vi "8-Test PingReq NoIdentifier.vi"() -> ()   [LabVIEW 2013]
uses:
  <vilib>/LabVIEW Open Source Project/MQTT Connection/MQTT_Connection/Connection/Connection.lvclass/Connection.ctl
  source/Server class/Server.lvclass/Server.ctl
  <vilib>/LabVIEW Open Source Project/MQTT Client/Client class/Client.lvclass/Client.ctl
  <vilib>/LabVIEW Open Source Project/MQTT Control Packets/Control Packets/PUBLISH/PUBLISH.lvclass
  source/Server class/Server.lvclass
  <vilib>/LabVIEW Open Source Project/MQTT Connection/MQTT_Base/Base Class/MQTT_Base.lvclass
  <vilib>/LabVIEW Open Source Project/MQTT Client/Client class/Client.lvclass
  <vilib>/LabVIEW Open Source Project/MQTT TCP Connection/MQTT_TCP/Connection/TCPConnection.lvclass
  <vilib>/LabVIEW Open Source Project/MQTT LocalQueue Connection/MQTT_LocalQueue/Connection/LocalQueueConnection.lvclass
  <vilib>/LabVIEW Open Source Project/MQTT Connection/MQTT_Connection/Connection/Connection.lvclass
  <vilib>/LabVIEW Open Source Project/MQTT Connection/MQTT_Base/DebuggingTerminal/DebuggingTerminal.lvclass
panel:
  out "#publish":i32
  out "error client source 2":errorcluster
  out "Published":bool
  out "ping time":i32
  out "#pings":i32
  out "PING FAILURE":bool
  out "Server responded":bool
  out "error server":errorcluster
  out "error client source":errorcluster
  out "NbConnections":u32
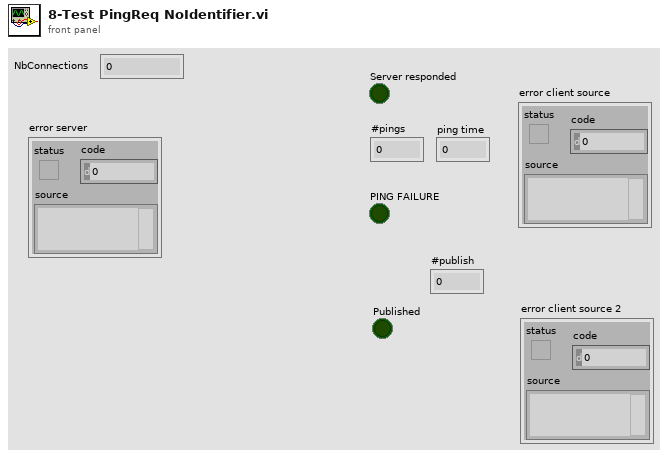
[diagram p1: front panel]
types:
  T1 = typedef "MQTT Client.lvlib/Client.lvclass/Public Events -- cluster.ctl" = cluster{"Connection Status":refnum<user-event>, "Connected":refnum<user-event>, "Application Message":refnum<user-event>}
  T2 = typedef "MQTT Server.lvlib/Server.lvclass/Public Events -- cluster.ctl" = cluster{"NbConnections":refnum<user-event>, "Client Event":refnum<user-event>}
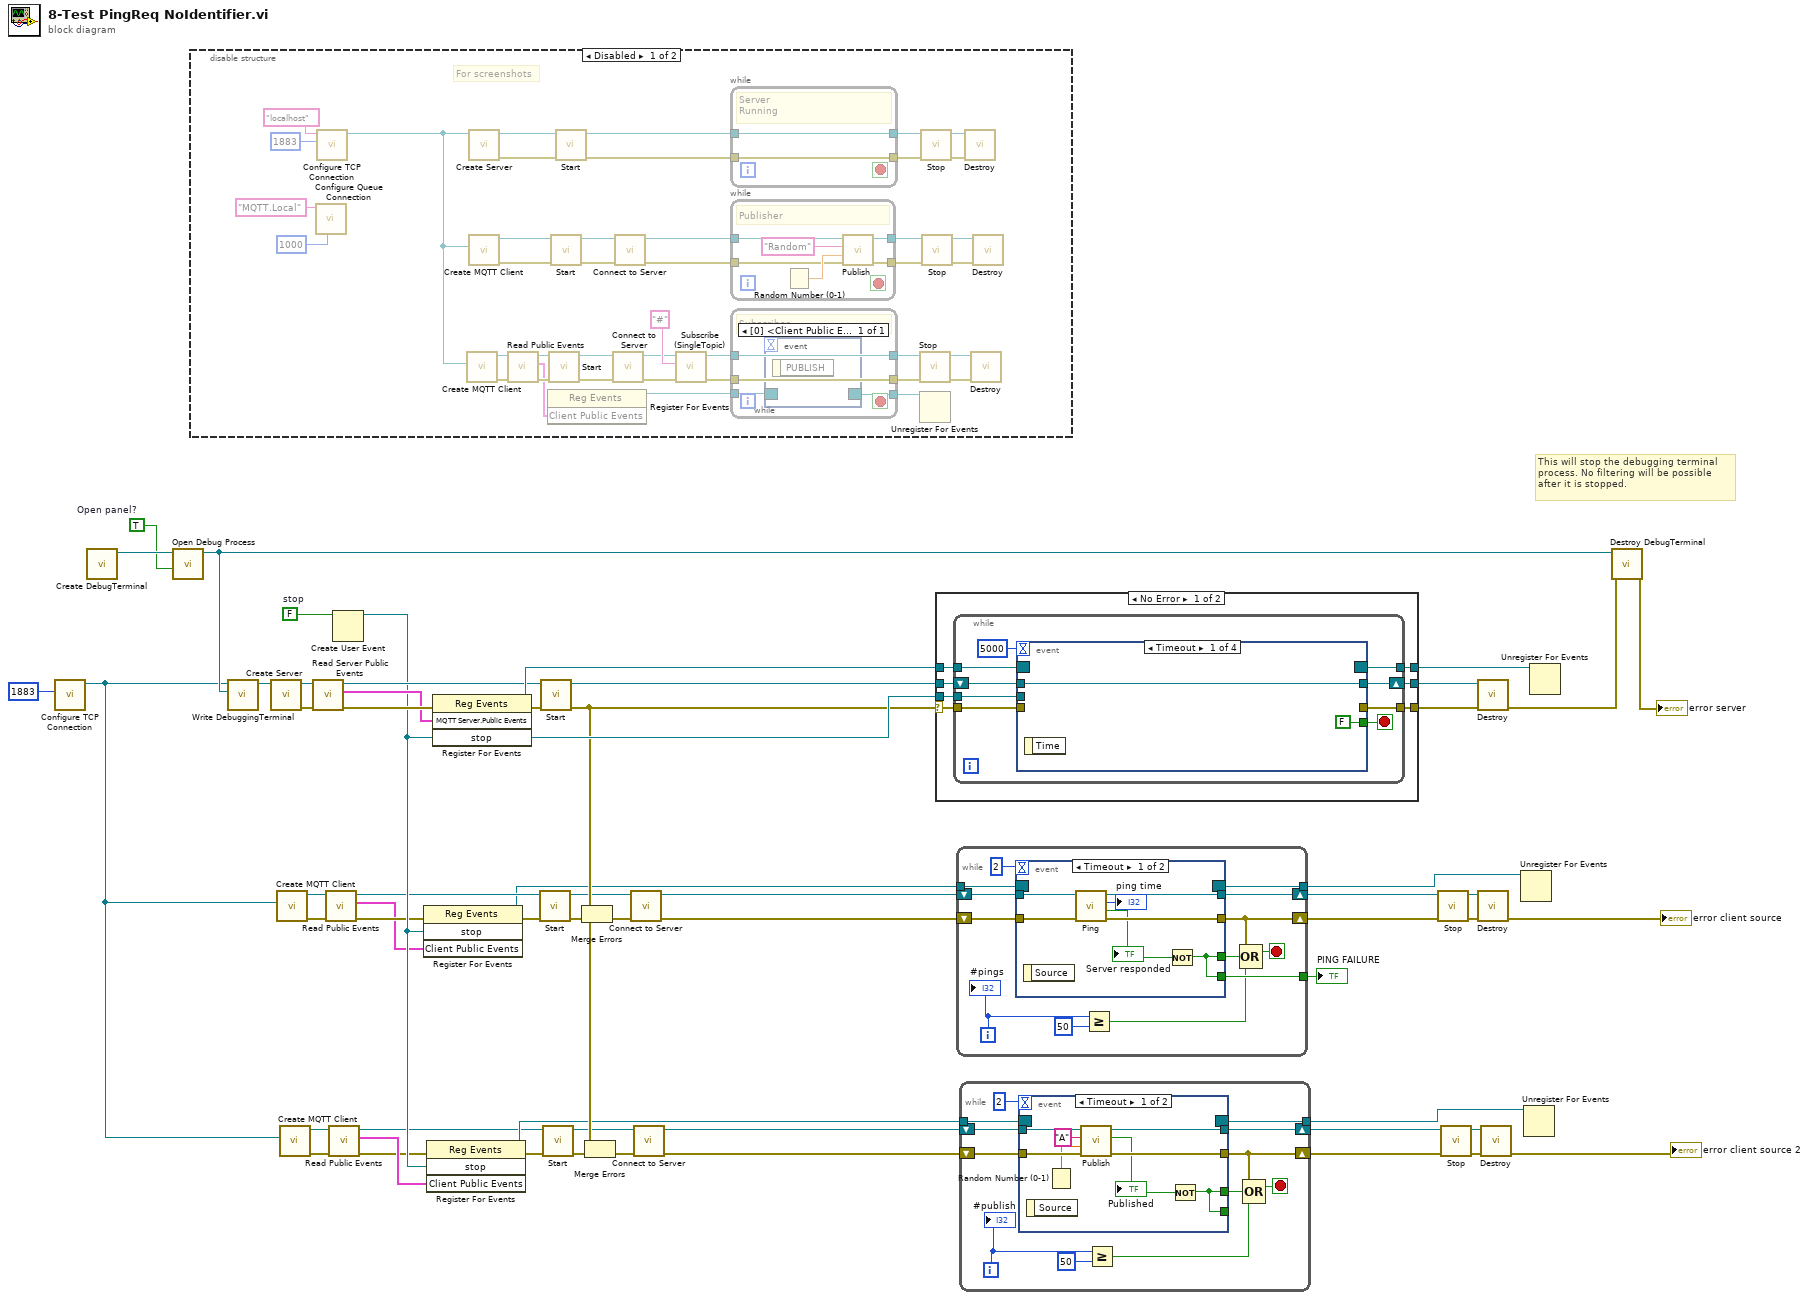
[diagram p0: block diagram]
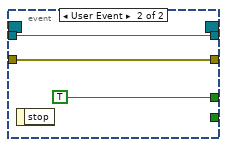
[diagram p2: hidden frame]
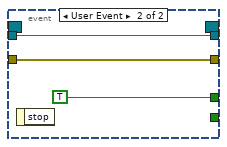
[diagram p3: hidden frame]
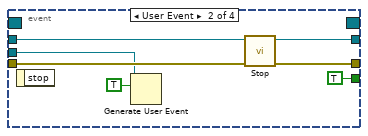
[diagram p5: hidden frame]
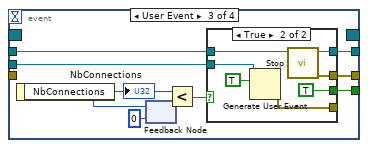
[diagram p6: hidden frame]
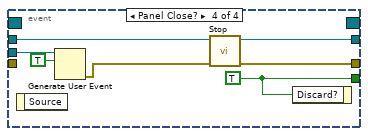
[diagram p8: hidden frame]
diagram:
  w1 = TRUE  # Open panel?
  w48 = FALSE  # stop
  # "This will stop the debugging terminal\nprocess. No filtering will be possible\nafter it is stopped."
  n1 = call <vilib>:"Configure TCP Connection.vi"("remote port (80)"=u16 1883) -> ("TCPConnection"=w5:refnum<class "TCPConnection.lvclass">)  [unwired: 9 in, 1 out]
  n2 = call <vilib>:"Create DebugTerminal.vi"() -> ("DebuggingTerminal out"=w9:refnum<class "DebuggingTerminal.lvclass">)  [unwired: 10 in, 1 out]
  n3 = call <vilib>:"Open Debug Process.vi"("Open panel?"=w1, "DebuggingTerminal in"=w9) -> ("DebuggingTerminal out"=w7:refnum<class "DebuggingTerminal.lvclass">)  [unwired: 8 in, 1 out]
  n4 = disable-structure shown="Disabled" {
    frame Disabled {
      # "For screenshots"
      n5 = call <vilib>:"Configure Queue Connection.vi"("timeout (500 ms)"=1000 ("timeout (100ms)"), "Queue Name"="MQTT.Local") -> ()  [unwired: 8 in, 2 out]
      n6 = call <vilib>:"Configure TCP Connection.vi"("remote port (80)"=u16 1883, "address (localhost)"="localhost" ("Topic Filter")) -> ("TCPConnection"=w63:refnum<class "TCPConnection.lvclass">)  [unwired: 8 in, 1 out]
      n7 = call <vilib>:"Create MQTT Client.vi"("Connection Configuration"=w63) -> ("error out"=w69:errorcluster, "Client out"=w71:refnum<class "Client.lvclass">)  [unwired: 9 in]
      n8 = call "Create Server.vi"("Connection Configuration"=w63) -> ("error out"=w94:errorcluster, "Server"=w93:refnum<class "Server.lvclass">)  [unwired: 9 in]
      n9 = call <vilib>:"Create MQTT Client.vi"("Connection Configuration"=w63) -> ("error out"=w91:errorcluster, "Client out"=w92:refnum<class "Client.lvclass">)  [unwired: 9 in]
      n10 = call <vilib>:"Read Public Events.vi"("error in (no error)"=w69, "Client in"=w71) -> ("error out"=w68:errorcluster, "Client Public Events"=w67:T1, "Client out"=w70:refnum<class "Client.lvclass">)  [unwired: 7 in]
      n11 = register-events(w67) -> (reference out=w66:refnum<event-registration>)  [unwired: 2 in, 1 out]
      n12 = call <vilib>:"Start.vi"("error in (no error)"=w68, "MQTT_Base in"=w70) -> ("error out"=w86:errorcluster, "MQTT_Base out"=w87:refnum<class "Client.lvclass">)  [unwired: 7 in, 1 out]
      n13 = call <vilib>:"Start.vi"("error in (no error)"=w91, "MQTT_Base in"=w92) -> ("error out"=w98:errorcluster, "MQTT_Base out"=w97:refnum<class "Client.lvclass">)  [unwired: 7 in, 1 out]
      n14 = call <vilib>:"Start.vi"("error in (no error)"=w94, "MQTT_Base in"=w93) -> ("error out"=w78:errorcluster, "MQTT_Base out"=w80:refnum<class "Server.lvclass">)  [unwired: 7 in, 1 out]
      n15 = call <vilib>:"Connect to Server.vi"("error in (no error)"=w86, "Client in"=w87) -> ("error out"=w74:errorcluster, "Client out"=w75:refnum<class "Client.lvclass">)  [unwired: 6 in, 2 out]
      n16 = call <vilib>:"Connect to Server.vi"("error in (no error)"=w98, "Client in"=w97) -> ("error out"=w82:errorcluster, "Client out"=w85:refnum<class "Client.lvclass">)  [unwired: 6 in, 2 out]
      n17 = call <vilib>:"Subscribe (SingleTopic).vi"("error in (no error)"=w74, "Topic Filter"="#", "MQTT_Base in"=w75) -> ("error out"=w72:errorcluster, "MQTT_Base out"=w73:refnum<class "Client.lvclass">)  [unwired: 6 in, 1 out]
      n18 = while {
        tunnel: [w112] -> w81
        tunnel: w80 -> [w112]
        tunnel: w78 -> [w111]
        tunnel: [w111] -> w79
        stop <- _ stop-if-true
        # "Server\nRunning"
      }
      n19 = while {
        tunnel: w85 -> [w108]
        tunnel: [w107] -> w84
        tunnel: [w106] -> w83
        tunnel: w82 -> [w105]
        stop <- _ stop-if-true
        # "Publisher"
        n20 = Random Number (0-1)() -> (number: 0 to 1=w110:dbl)
        n21 = call <vilib>:"Publish.vi"("error in (no error)"=w105, "Payload"=w110, "Topic Name (empty: Payload name)"="Random", "Client in"=w108) -> ("error out"=w106:errorcluster, "Client out"=w107:refnum<class "Client.lvclass">)  [unwired: 5 in, 1 out]
      }
      n22 = while {
        tunnel: [w104] -> w76
        tunnel: w73 -> [w104]
        tunnel: w72 -> [w103]
        tunnel: [w103] -> w77
        tunnel: w66 -> [w102]
        tunnel: [w101] -> w65
        stop <- _ stop-if-true
        # "Subscriber"
        n23 = event shown="[0] <Client Public Events.Application Message>: User Event" {
          selector: w102 -> [_]
          dyn-events: [_] -> w101
          timeout: _ -> [_]
          event User Event {
            n24 = event-data() -> ()  [unwired: 1 in, 1 out]
          }
        }
      }
      n25 = call <vilib>:"Stop.vi"("error in (no error)"=w77, "MQTT_Base in"=w76) -> ("error out"=w89:errorcluster, "MQTT_Base out"=w90:refnum<class "Client.lvclass">)  [unwired: 7 in, 1 out]
      n26 = Unregister For Events(event registration refnum=w65) -> ()  [unwired: 1 in, 1 out]
      n27 = call <vilib>:"Stop.vi"("error in (no error)"=w79, "MQTT_Base in"=w81) -> ("error out"=w100:errorcluster, "MQTT_Base out"=w99:refnum<class "Server.lvclass">)  [unwired: 7 in, 1 out]
      n28 = call <vilib>:"Stop.vi"("error in (no error)"=w83, "MQTT_Base in"=w84) -> ("error out"=w96:errorcluster, "MQTT_Base out"=w95:refnum<class "Client.lvclass">)  [unwired: 7 in, 1 out]
      n29 = call <vilib>:"Destroy.vi"("error in (no error)"=w100, "MQTT_Base in"=w99) -> ()  [unwired: 8 in, 2 out]
      n30 = call <vilib>:"Destroy.vi"("error in (no error)"=w89, "MQTT_Base in"=w90) -> ()  [unwired: 8 in, 2 out]
      n31 = call <vilib>:"Destroy.vi"("error in (no error)"=w96, "MQTT_Base in"=w95) -> ()  [unwired: 8 in, 2 out]
    }
    frame Enabled {
    }
  }
  n32 = call <vilib>:"Write DebuggingTerminal.vi"("DebuggingTerminal"=w7, "Connection in"=w5) -> ("Connection out"=w4:refnum<class "TCPConnection.lvclass">)  [unwired: 9 in]
  n33 = call "Create Server.vi"("Connection Configuration"=w4) -> ("error out"=w57:errorcluster, "Server"=w58:refnum<class "Server.lvclass">)  [unwired: 9 in]
  n34 = call <vilib>:"Create MQTT Client.vi"("Connection Configuration"=w5) -> ("error out"=w44:errorcluster, "Client out"=w43:refnum<class "Client.lvclass">)  [unwired: 9 in]
  n35 = call <vilib>:"Create MQTT Client.vi"("Connection Configuration"=w5) -> ("error out"=w12:errorcluster, "Client out"=w13:refnum<class "Client.lvclass">)  [unwired: 9 in]
  n36 = call "Read Server Public Events.vi"("error in (no error)"=w57, "Server in"=w58) -> ("error out"=w56:errorcluster, "MQTT Server.Public Events"=w55:T2, "Server out"=w52:refnum<class "Server.lvclass">)  [unwired: 7 in]
  n37 = call <vilib>:"Read Public Events.vi"("error in (no error)"=w44, "Client in"=w43) -> ("error out"=w36:errorcluster, "Client Public Events"=w32:T1, "Client out"=w42:refnum<class "Client.lvclass">)  [unwired: 7 in]
  n38 = call <vilib>:"Read Public Events.vi"("error in (no error)"=w12, "Client in"=w13) -> ("error out"=w20:errorcluster, "Client Public Events"=w24:T1, "Client out"=w14:refnum<class "Client.lvclass">)  [unwired: 7 in]
  n39 = Create User Event(user event datatype=w48) -> (user event=w47:refnum<user-event>)  [unwired: 1 in, 1 out]
  n40 = register-events(error in=w36, w47, w32) -> (reference out=w34:refnum<event-registration>, error out=w35:errorcluster)  [unwired: 1 in]
  n41 = register-events(error in=w20, w47, w24) -> (reference out=w22:refnum<event-registration>, error out=w21:errorcluster)  [unwired: 1 in]
  n42 = register-events(error in=w56, w55, w47) -> (reference out=w54:refnum<event-registration>, error out=w50:errorcluster)  [unwired: 1 in]
  n43 = call <vilib>:"Start.vi"("error in (no error)"=w35, "MQTT_Base in"=w42) -> ("error out"=w40:errorcluster, "MQTT_Base out"=w41:refnum<class "Client.lvclass">)  [unwired: 7 in, 1 out]
  n44 = call <vilib>:"Start.vi"("error in (no error)"=w50, "MQTT_Base in"=w52) -> ("error out"=w46:errorcluster, "MQTT_Base out"=w51:refnum<class "Server.lvclass">)  [unwired: 7 in, 1 out]
  n45 = call <vilib>:"Start.vi"("error in (no error)"=w21, "MQTT_Base in"=w14) -> ("error out"=w16:errorcluster, "MQTT_Base out"=w15:refnum<class "Client.lvclass">)  [unwired: 7 in, 1 out]
  n46 = Merge Errors(w46, w40) -> (w45:errorcluster)
  n47 = Merge Errors(w46, w16) -> (w11:errorcluster)
  n48 = call <vilib>:"Connect to Server.vi"("error in (no error)"=w45, "Client in"=w41) -> ("error out"=w29:errorcluster, "Client out"=w30:refnum<class "Client.lvclass">)  [unwired: 6 in, 2 out]
  n49 = call <vilib>:"Connect to Server.vi"("error in (no error)"=w11, "Client in"=w15) -> ("error out"=w27:errorcluster, "Client out"=w26:refnum<class "Client.lvclass">)  [unwired: 6 in, 2 out]
  n50 = case shown="No Error" w46 {
    selector: w46 -> [w113 w162]
    tunnel: w51 -> [w119 w164]
    tunnel: [w118 w164] -> w59
    tunnel: w54 -> [w117 w163]
    tunnel: [w116 w163] -> w53
    tunnel: [w115 w162] -> w49
    tunnel: w47 -> [w114 _]
    frame No Error {
      n51 = while {
        shift-right: [w125] -> w118
        shift-left: w119 -> [w127]
        tunnel: w117 -> [w124]
        tunnel: [w123] -> w116
        tunnel: [w122] -> w115
        tunnel: w114 -> [w121]
        tunnel: w113 -> [w120]
        stop <- w126 stop-if-true
        n52 = event shown="[0] Timeout" {
          selector: w124 -> [_ _ _ _]
          dyn-events: [_ _ _ _] -> w123
          timeout: 5000 -> [_ _ _ _]
          tunnel: w127 -> [w130 w137 w143 w161]
          tunnel: [FALSE ("Discard?") TRUE ("Discard?") w139 w160] -> w126
          tunnel: [w130 w136 w142 w159] -> w125
          tunnel: [_ w135 w141 w158] -> w122
          tunnel: w121 -> [_ w131 w138 w157]
          tunnel: w120 -> [_ w133 _ _]
          event Timeout {
            n53 = event-data() -> ()  [unwired: 1 in, 1 out]
          }
          event User Event {
            n54 = event-data() -> ()  [unwired: 1 in, 1 out]
            n55 = Generate User Event(user event=w131, event data cluster=TRUE ("event data")) -> ()  [unwired: 2 in, 2 out]
            n56 = call <vilib>:"Stop.vi"("error in (no error)"=w133, "MQTT_Base in"=w137) -> ("error out"=w135:errorcluster, "MQTT_Base out"=w136:refnum<class "Server.lvclass">)  [unwired: 7 in, 1 out]
          }
          event User Event {
            n57 = event-data() -> ("NbConnections"=w145:u32)  [unwired: 1 in]
            "NbConnections" <- w145
            n58 = feedback #1(u32 0 ("NbConnections")) -> (w144:u32)
            n59 = feedback-in #1(w145) -> ()
            n60 = Less?(x=w145, y=w144) -> (x < y?=w140:bool)
            n61 = case shown="True" w140 {
              tunnel: w143 -> [w147 w154]
              tunnel: [w147 w153] -> w142
              tunnel: [_ w152] -> w141
              tunnel: [_ TRUE] -> w139
              tunnel: w138 -> [_ w149]
              tunnel: [_ w148] -> _
              frame False {
              }
              frame True {
                n62 = Generate User Event(user event=w149, event data cluster=TRUE ("event data")) -> (error out=w148:errorcluster)  [unwired: 2 in, 1 out]
                n63 = call <vilib>:"Stop.vi"("MQTT_Base in"=w154) -> ("error out"=w152:errorcluster, "MQTT_Base out"=w153:refnum<class "Server.lvclass">)  [unwired: 8 in, 1 out]
              }
            }
          }
          event Panel Close? {
            w160 = TRUE ("Discard?")
            n64 = event-data() -> ()  [unwired: 1 in, 1 out]
            n65 = Generate User Event(user event=w157, event data cluster=TRUE ("event data")) -> (error out=w155:errorcluster)  [unwired: 2 in, 1 out]
            n66 = call <vilib>:"Stop.vi"("error in (no error)"=w155, "MQTT_Base in"=w161) -> ("error out"=w158:errorcluster, "MQTT_Base out"=w159:refnum<class "Server.lvclass">)  [unwired: 7 in, 1 out]
            n67 = event-data("Discard?"=w160) -> ()  [unwired: 1 in, 1 out]
          }
        }
      }
    }
    frame Error {
    }
  }
  n68 = while {
    shift-right: [w176] -> w39
    shift-left: w30 -> [w177]
    shift-right: [w169] -> w33
    shift-left: w29 -> [w175]
    tunnel: w34 -> [w173]
    tunnel: [w171] -> w31
    tunnel: [w168] -> w28
    i -> [w167]
    stop <- w174 stop-if-true
    n69 = event shown="[0] Timeout" {
      selector: w173 -> [_ _]
      dyn-events: [_ _] -> w171
      timeout: 2 -> [_ _]
      tunnel: w177 -> [w184 w185]
      tunnel: [w183 w185] -> w176
      tunnel: w175 -> [w181 w186]
      tunnel: [w182 w186] -> w169
      tunnel: [w179 TRUE] -> w172
      tunnel: [w179 _] -> w168
      event Timeout {
        n70 = event-data() -> ()  [unwired: 1 in, 1 out]
        n71 = call <vilib>:"Ping.vi"("error in (no error)"=w181, "Client in"=w184) -> ("error out"=w182:errorcluster, "Server responded"=w180:bool, "ping time"=→"ping time":i32, "Client out"=w183:refnum<class "Client.lvclass">)  [unwired: 6 in]
        "Server responded" <- w180
        n72 = Not(x=w180) -> (.not. x?=w179:bool)
      }
      event User Event {
        n73 = event-data() -> ()  [unwired: 1 in, 1 out]
      }
    }
    n74 = Greater Or Equal?(x=w167, y=50) -> (x >= y?=w165:bool)
    n75 = Compound Arithmetic op=OR(w169, w172, w165) -> (w174:bool)
    "#pings" <- w167
  }
  "PING FAILURE" <- w28
  n76 = while {
    shift-right: [w198] -> w17
    shift-left: w26 -> [w199]
    shift-right: [w191] -> w23
    shift-left: w27 -> [w197]
    tunnel: w22 -> [w195]
    tunnel: [w193] -> w25
    i -> [w188]
    stop <- w196 stop-if-true
    n77 = event shown="[0] Timeout" {
      selector: w195 -> [_ _]
      dyn-events: [_ _] -> w193
      timeout: 2 -> [_ _]
      tunnel: w199 -> [w206 w208]
      tunnel: [w205 w208] -> w198
      tunnel: w197 -> [w204 w209]
      tunnel: [w203 w209] -> w191
      tunnel: [w207 TRUE] -> w194
      tunnel: [w207 _] -> _
      event Timeout {
        n78 = event-data() -> ()  [unwired: 1 in, 1 out]
        n79 = Random Number (0-1)() -> (number: 0 to 1=w200:dbl)
        n80 = call <vilib>:"Publish.vi"("error in (no error)"=w204, "Payload"=w200, "Topic Name (empty: Payload name)"="A", "Client in"=w206) -> ("error out"=w203:errorcluster, "Published"=w202:bool, "Client out"=w205:refnum<class "Client.lvclass">)  [unwired: 5 in]
        "Published" <- w202
        n81 = Not(x=w202) -> (.not. x?=w207:bool)
      }
      event User Event {
        n82 = event-data() -> ()  [unwired: 1 in, 1 out]
      }
    }
    n83 = Greater Or Equal?(x=w188, y=50) -> (x >= y?=w189:bool)
    n84 = Compound Arithmetic op=OR(w191, w194, w189) -> (w196:bool)
    "#publish" <- w188
  }
  n85 = call <vilib>:"Stop.vi"("error in (no error)"=w33, "MQTT_Base in"=w39) -> ("error out"=w37:errorcluster, "MQTT_Base out"=w38:refnum<class "Client.lvclass">)  [unwired: 7 in, 1 out]
  n86 = call <vilib>:"Stop.vi"("error in (no error)"=w23, "MQTT_Base in"=w17) -> ("error out"=w19:errorcluster, "MQTT_Base out"=w18:refnum<class "Client.lvclass">)  [unwired: 7 in, 1 out]
  n87 = call <vilib>:"Destroy.vi"("error in (no error)"=w49, "MQTT_Base in"=w59) -> ("error out"=w3:errorcluster)  [unwired: 8 in, 1 out]
  n88 = call <vilib>:"Destroy.vi"("error in (no error)"=w37, "MQTT_Base in"=w38) -> ("error out"=→"error client source":errorcluster)  [unwired: 8 in, 1 out]
  n89 = call <vilib>:"Destroy.vi"("error in (no error)"=w19, "MQTT_Base in"=w18) -> ("error out"=→"error client source 2":errorcluster)  [unwired: 8 in, 1 out]
  n90 = Unregister For Events(event registration refnum=w31) -> ()  [unwired: 1 in, 1 out]
  n91 = Unregister For Events(event registration refnum=w25) -> ()  [unwired: 1 in, 1 out]
  n92 = Unregister For Events(event registration refnum=w53) -> ()  [unwired: 1 in, 1 out]
  n93 = call <vilib>:"Destroy DebugTerminal.vi"("error in (no error)"=w3, "DebuggingTerminal in"=w7) -> ("error out"=→"error server":errorcluster)  [unwired: 8 in, 1 out]
